vi "visa_write_test.vi"() -> ()   [LabVIEW 2013]
uses:
  <vilib>/Instr/_visa.llb/VISA Configure Serial Port (Instr).vi
panel:
  out "读取缓冲区":string
  out "返回数":u32
  in  "写入缓冲区":string="#1GC2\\r\\n"
  in  "baud rate (9600)":u32=115200 caption="波特率(9600)"
  in  "VISA resource name":refnum<visa-resource-name> caption="VISA资源名称"
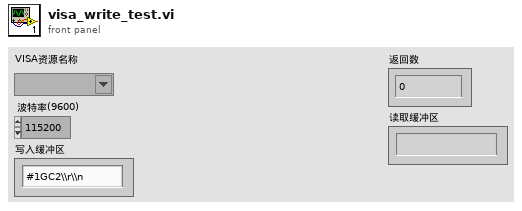
[diagram p1: front panel]
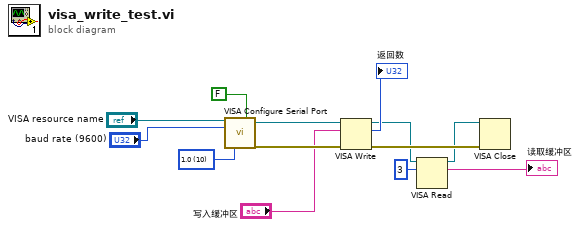
[diagram p0: block diagram]
diagram:
  w2 = u16 10 items=["1.0"=10, "1.5"=15, "2.0"=20] ("stop bits (10: 1 bit)")
  n1 = call-poly "VISA Configure Serial Port"("VISA resource name"="VISA resource name", "Enable Termination\nChar (T)"=FALSE ("Enable Termination\nChar (T)"), "baud rate (9600)"="baud rate (9600)", "stop bits (10: 1 bit)"=w2) -> ("VISA resource name out"=w11:refnum<visa-resource-name>, "error out"=w10:errorcluster)  [unwired: 10 in]
  n2 = VISA Write(VISA resource name=w11, write buffer="写入缓冲区", error in (no error)=w10) -> (VISA resource name out=w6:refnum<visa-resource-name>, return count=→"返回数":u32, error out=w9:errorcluster)
  n3 = VISA Read(VISA resource name=w6, byte count=u32 3 ("字节总数")) -> (VISA resource name out=w5:refnum<visa-resource-name>, read buffer=→"读取缓冲区":string)  [unwired: 1 in, 2 out]
  n4 = VISA Close(VISA resource name=w5, error in (no error)=w9) -> ()  [unwired: 1 out]
